vi "SetWindowParent.vi"(8 "No Error":errorcluster, 10 "Parent [SDL_Window *] (0: No Parent)":i64 format="%.0x", 11 "Window [SDL_Window *]":i64 format="%.0x") -> (0 "Error Out":errorcluster)   [LabVIEW 2024, in "SDL3.lvlib" / "Video.lvlib"]
doc: "<B>Summary</B>\nSet the window as a child of a parent window.\n\n<B>Remarks</B>\nIf the window is already the child of an existing window, it will be reparented to the new owner. Setting the parent window to NULL unparents the window and removes child window status.\n\nIf a parent window is hidden or destroyed, the operation will be recursively applied to child windows. Child windows hidden with the parent that did not have their hidden status explicitly set will be restored when the parent is shown.\n\nAttempting to set the parent of a window that is currently in the modal state will fail. Use <B>SDL_SetWindowModal()</B> to cancel the modal status before attempting to change the parent.\n\nPopup windows cannot change parents and attempts to do so will fail.\n\nSetting a parent window that is currently the sibling or descendent of the child window results in undefined behavior."
uses:
  Video.lvlib
  Lib/Win32/SDL3.dll
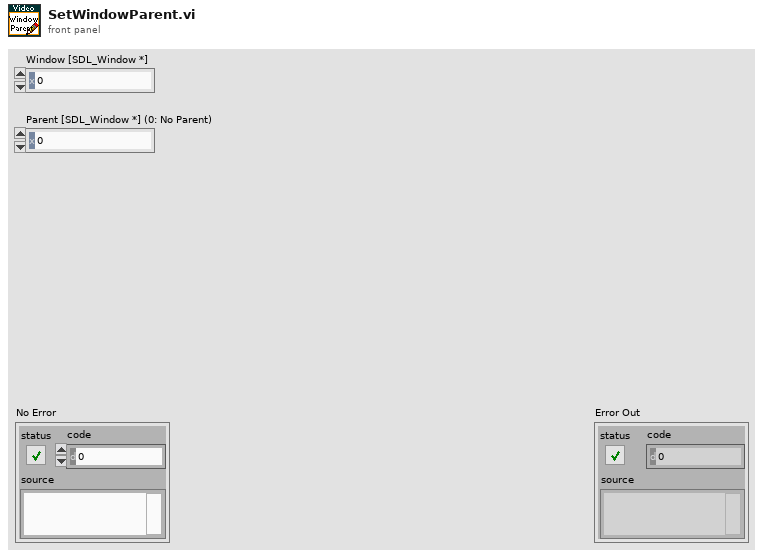
[diagram p1: front panel]
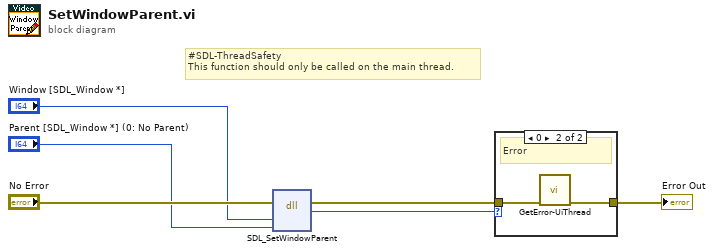
[diagram p0: block diagram]
diagram:
  # "#SDL-ThreadSafety\nThis function should only be called on the main thread."
  n1 = dll-call lib="C:/Users/Thomas/Documents/Projects/LV-SDL3/Lib/Win32/SDL3.dll" fn="SDL_SetWindowParent"(error in="No Error", "window"="Window [SDL_Window *]", "parent"="Parent [SDL_Window *] (0: No Parent)") -> (error out=w3:errorcluster, "return type"=w2:i32)  [unwired: 4 in, 1 out]
  n2 = case shown="0" w2 {
    tunnel: w3 -> [w7 w9]
    tunnel: [w7 w8] -> w5
    frame Default {
      # "Ok"
    }
    frame 0 {
      # "Error"
      n3 = call "GetError-UiThread.vi"("No Error"=w9) -> ("error out"=w8:errorcluster)  [unwired: 10 in]
    }
  }
  "Error Out" <- w5
